vi "历史查询数据.vi"() -> ()   [LabVIEW 2019]
panel:
  out "用户名":string
  out "错误输出 2":errorcluster caption="错误输出"
  out "用户类型":string
  out "错误输出":errorcluster
  out "error out 6":errorcluster
  out "error out 5":errorcluster
  out "Row":i32
  out "Column":i32
  out "error out 7":errorcluster
  out "当前选择的记录为":string
  in  "导出文件":bool
  in  "删除记录":bool
  out "车牌查询数据":string[][](table)
  in  "返回":bool
  # "欢迎查询识别记录"
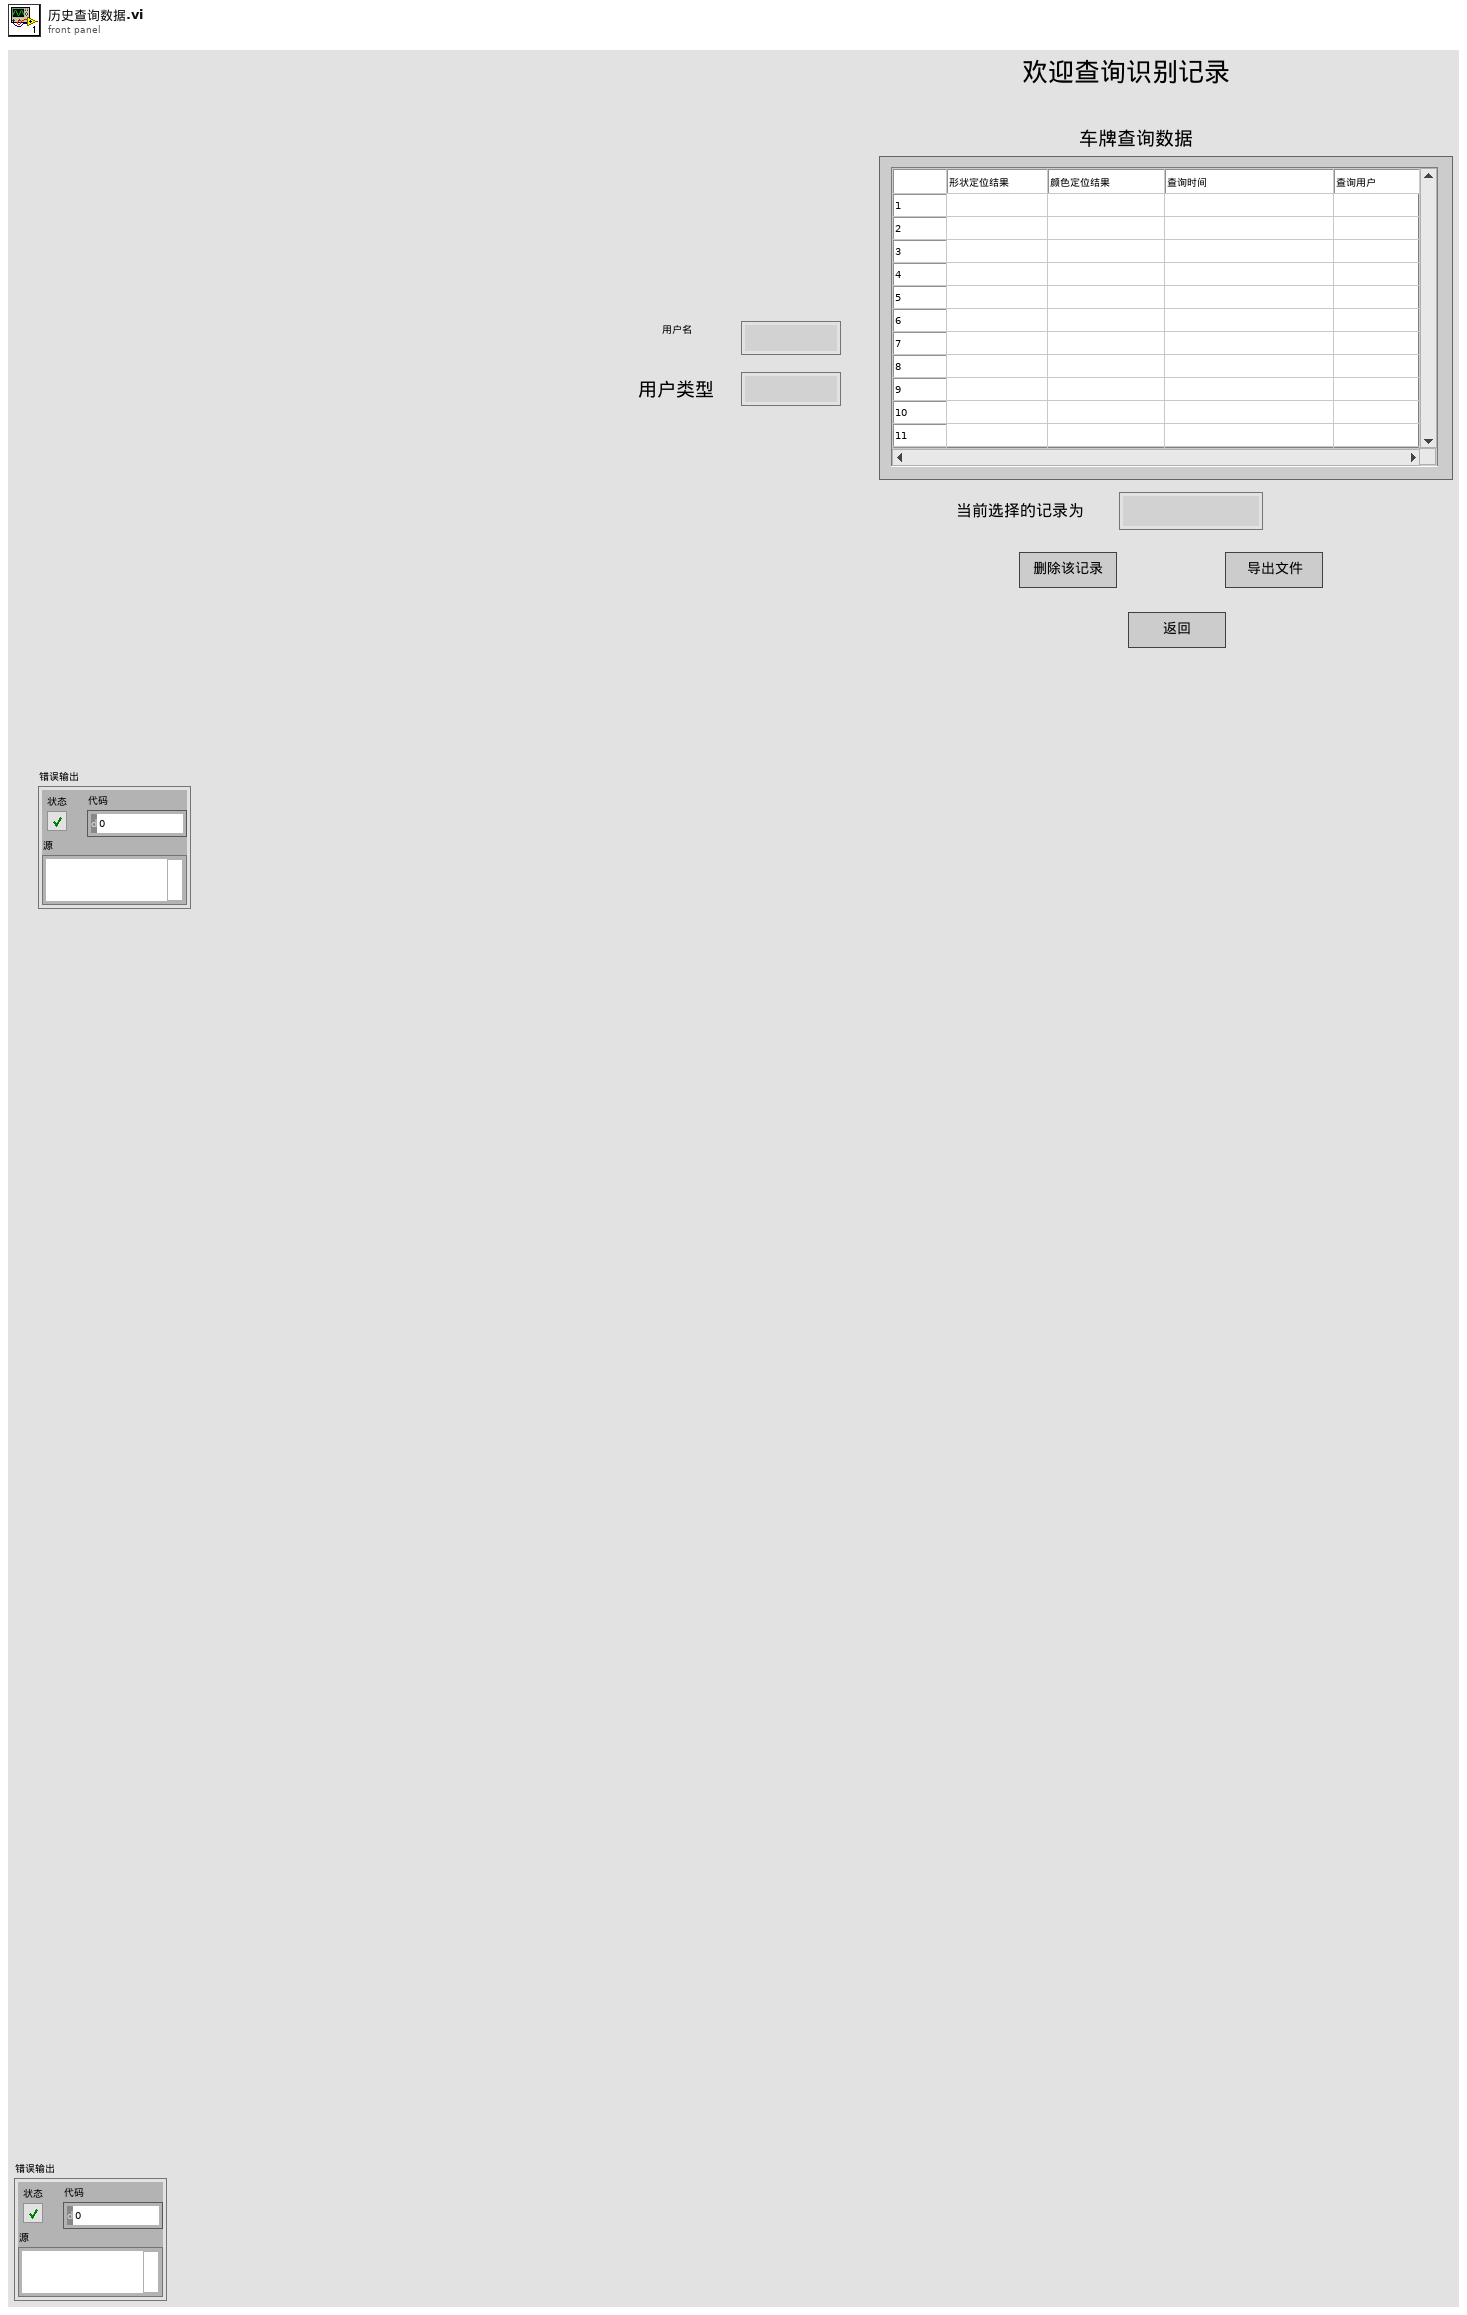
[diagram p1: front panel]
types:
  T1 = typedef "LVPoint32TypeDef.ctl" = cluster{"Horizontal":i32, "Vertical":i32}
  T2 = typedef "LVRowAndColumnTypeDef.ctl" = cluster{"Row":i32, "Column":i32}
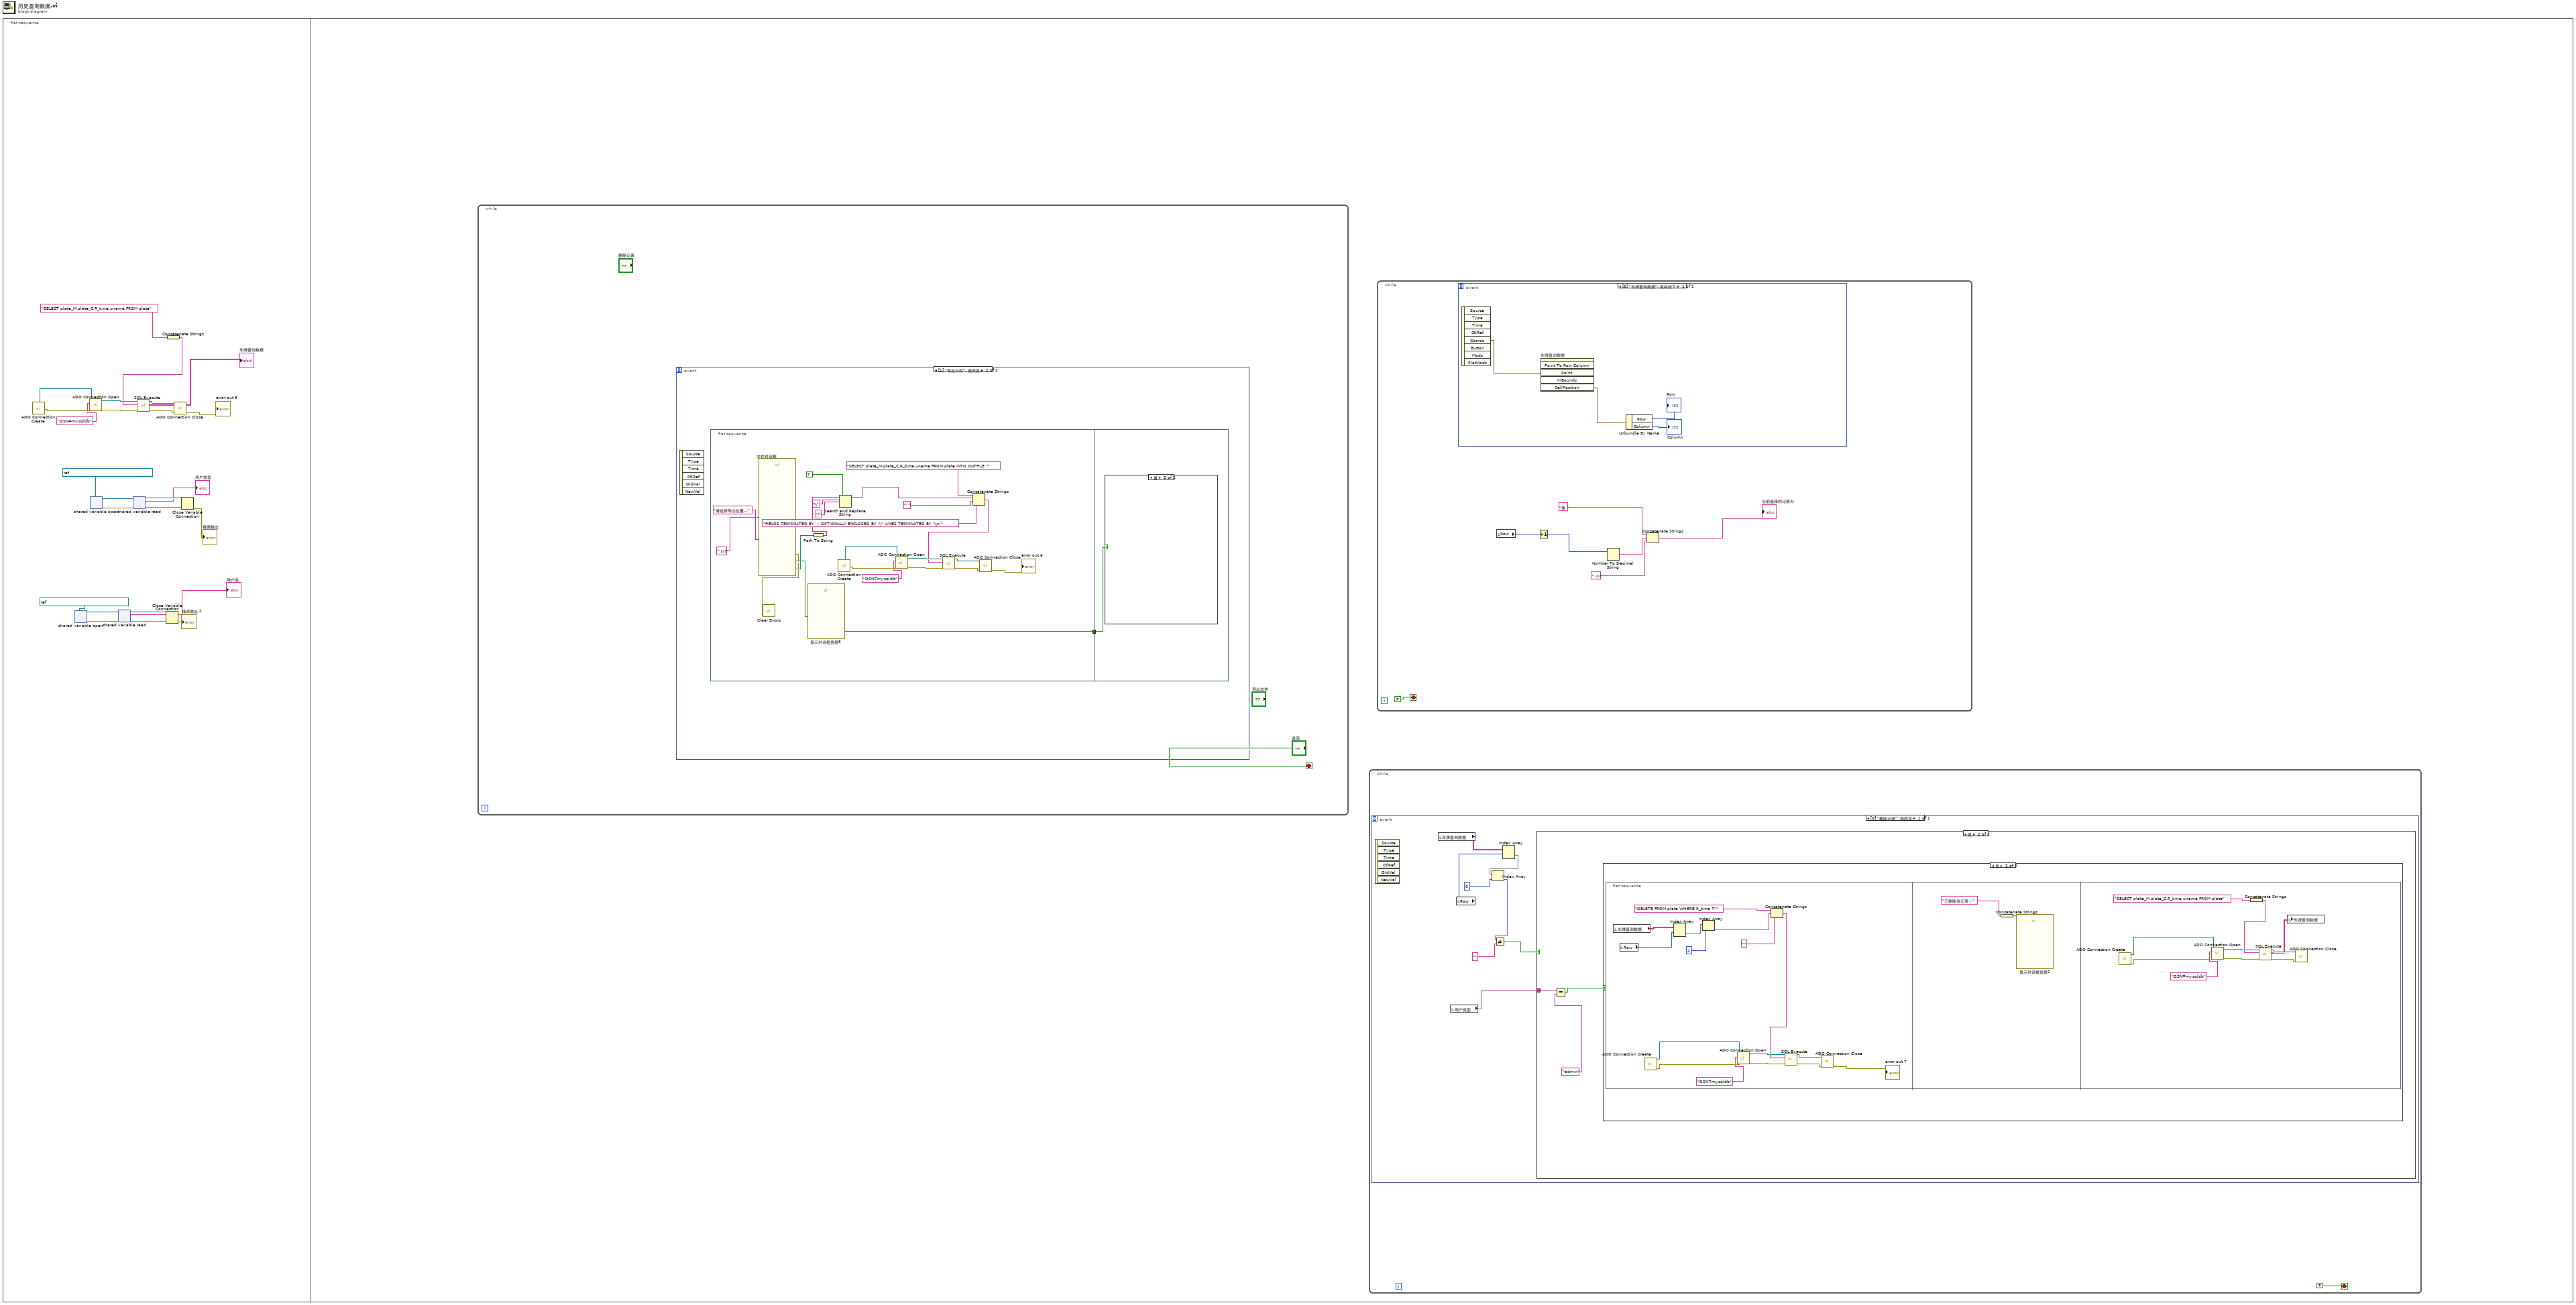
[diagram p0: block diagram]
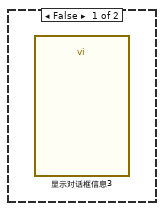
[diagram p2: hidden frame]
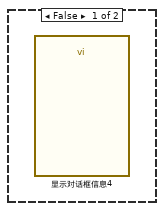
[diagram p3: hidden frame]
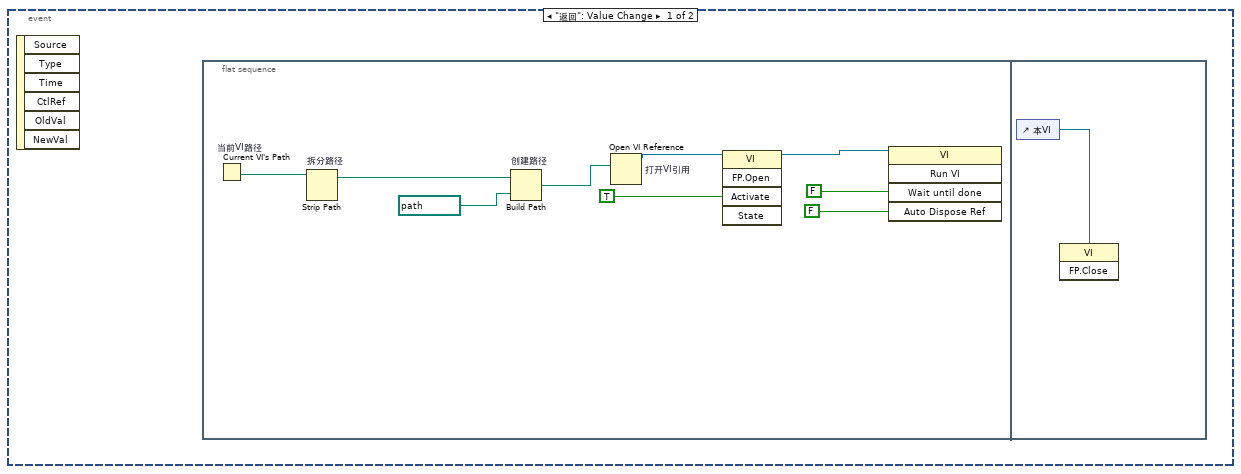
[diagram p4: hidden frame]
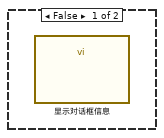
[diagram p5: hidden frame]
diagram:
  n1 = flat-sequence {
    frame #0 {
      n2 = call <userlib>:"ADO Connection Create.vi"() -> ("error out"=w20:errorcluster, "ADODB._Connection Out"=w19:refnum<k7>)  [unwired: 10 in]
      n3 = shared-variable-open(refnum<k21> "ni.var.psp://我的电脑/登录/登录用户" ("共享变量引用句柄输入")) -> (w3:refnum<k21>, w4:errorcluster)  [unwired: 2 in]
      n4 = call <userlib>:"ADO Connection Open.vi"("error in (no error)"=w20, "ConnectionString"="DSN=mysqldb", "ADODB._Connection In"=w19) -> ("error out"=w21:errorcluster, "ADODB._Connection Out"=w25:refnum<k7>)  [unwired: 7 in]
      n5 = shared-variable-open(refnum<k21> "ni.var.psp://localhost/登录/用户类型" ("共享变量引用句柄输入")) -> (w14:refnum<k21>, w13:errorcluster)  [unwired: 2 in]
      n6 = shared-variable-read(w3, w4) -> (w5:refnum<k21>, w6:errorcluster, →"用户名":string)  [unwired: 1 out]
      n7 = shared-variable-read(w14, w13) -> (w12:refnum<k21>, w11:errorcluster, →"用户类型":string)  [unwired: 1 out]
      n8 = Close Variable Connection(8:w6, 11:w5) -> (0:→"错误输出 2":errorcluster)
      n9 = Concatenate Strings("SELECT plate_M,plate_C,R_time,uname FROM plate") -> (w16:string)
      n10 = call <userlib>:"SQL Execute.vi"("error in (no error)"=w21, "Command Text"=w16, "ADODB._Connection In"=w25) -> ("error out"=w23:errorcluster, "Data"=→"车牌查询数据":string[][], "ADODB._Connection Out"=w24:refnum<k7>)  [unwired: 5 in, 1 out]
      n11 = call <userlib>:"ADO Connection Close.vi"("error in (no error)"=w23, "ADODB._Connection In"=w24) -> ("error out"=→"error out 5":errorcluster)  [unwired: 8 in, 1 out]
      n12 = Close Variable Connection(8:w11, 11:w12) -> (0:→"错误输出":errorcluster)
    }
    frame #1 {
      n13 = while {
        stop <- "返回" stop-if-true
        n14 = event shown="[1] \"导出文件\": 值改变" {
          selector: _ -> [_ _]
          dyn-events: _ -> [_ _]
          timeout: _ -> [_ _]
          event "返回": Value Change {
            n15 = event-data() -> ()  [unwired: 1 in, 6 out]
            n16 = flat-sequence {
              frame #0 {
                n17 = Current VI's Path "当前VI路径"() -> (path=w79:path)
                n18 = Strip Path "拆分路径"(path=w79) -> (stripped path=w78:path)  [unwired: 1 out]
                n19 = Build Path "创建路径"(base path=w78, name or relative path=path "登陆后.vi") -> (appended path=w81:path)
                n20 = Open VI Reference "打开VI引用"(vi path=w81) -> (vi reference=w80:refnum<vi>)  [unwired: 5 in, 1 out]
                n21 = invoke class="VI" method="FP.Open"(reference=w80, "Activate"=TRUE) -> (reference out=w84:refnum<vi>)  [unwired: 3 in, 4 out]
                n22 = invoke class="VI" method="Run VI"(reference=w84, "Wait until done"=FALSE, "Auto Dispose Ref"=FALSE) -> ()  [unwired: 2 in, 5 out]
              }
              frame #1 {
                n23 = control-ref of="本VI"() -> (w87:refnum<vi>)
                n24 = invoke class="VI" method="FP.Close"(reference=w87) -> ()  [unwired: 2 in, 3 out]
              }
            }
          }
          event "导出文件": Value Change {
            n25 = event-data() -> ()  [unwired: 1 in, 6 out]
            n26 = flat-sequence {
              tunnel: [w90] -> w88
              tunnel: w88 -> [w112]
              frame #0 {
                n27 = call "文件对话框"("prompt"="请选择导出位置...", "pattern (all files)"=".txt") -> ("selected path"=w98:path, "cancelled"=w91:bool, "error out"=w89:errorcluster)  [unwired: 10 in, 1 out]
                n28 = call <vilib>:"Clear Errors.vi"("error in (no error)"=w89) -> ()  [unwired: 5 in, 2 out]
                n29 = call "显示对话框信息5"("Enable"=w91) -> ("确定"=w90:bool)  [unwired: 9 in, 1 out]
                n30 = Path To String(path=w98) -> (string=w94:string)
                n31 = call <userlib>:"ADO Connection Create.vi"() -> ("error out"=w104:errorcluster, "ADODB._Connection Out"=w103:refnum<k7>)  [unwired: 10 in]
                n32 = Search and Replace String(replace all?=TRUE, input string=w94, search string="\\", replace string="/") -> (result string=w93:string)  [unwired: 4 in, 3 out]
                n33 = call <userlib>:"ADO Connection Open.vi"("error in (no error)"=w104, "ConnectionString"="DSN=mysqldb", "ADODB._Connection In"=w103) -> ("error out"=w105:errorcluster, "ADODB._Connection Out"=w109:refnum<k7>)  [unwired: 7 in]
                n34 = Concatenate Strings("SELECT plate_M,plate_C,R_time,uname FROM plate INTO OUTFILE '", w93, "' ", "FIELDS TERMINATED BY ',' OPTIONALLY ENCLOSED BY '\"' LINES TERMINATED BY '\\n'") -> (w100:string)
                n35 = call <userlib>:"SQL Execute.vi"("error in (no error)"=w105, "Command Text"=w100, "ADODB._Connection In"=w109) -> ("error out"=w107:errorcluster, "ADODB._Connection Out"=w108:refnum<k7>)  [unwired: 5 in, 2 out]
                n36 = call <userlib>:"ADO Connection Close.vi"("error in (no error)"=w107, "ADODB._Connection In"=w108) -> ("error out"=→"error out 6":errorcluster)  [unwired: 8 in, 1 out]
              }
              frame #1 {
                n37 = case shown="真" w112 {
                  frame False {
                    n38 = call "显示对话框信息"() -> ()  [unwired: 10 in, 2 out]
                  }
                  frame True {
                  }
                }
              }
            }
          }
        }
      }
      n39 = while {
        stop <- FALSE stop-if-true
        n40 = event shown="[0] \"删除记录\": 值改变" {
          selector: _ -> [_]
          dyn-events: _ -> [_]
          timeout: _ -> [_]
          event "删除记录": Value Change {
            n41 = event-data() -> ()  [unwired: 1 in, 6 out]
            n42 = local read "车牌查询数据"() -> (w33:string[][])
            n43 = local read "用户类型"() -> (w27:string)
            n44 = local read "Row"() -> (w32:i32)
            n45 = Index Array(array=w33, index (row)=w32) -> (element=w31:string[])  [unwired: 1 in]
            n46 = Index Array(array=w31, index=0) -> (element=w28:string)
            n47 = Not Equal?(x=w28, y="") -> (x != y?=w29:bool)
            n48 = case shown="真" w29 {
              tunnel: w27 -> [_ w37]
              frame False {
                n49 = call "显示对话框信息3"() -> ()  [unwired: 10 in, 2 out]
              }
              frame True {
                n50 = Equal?(x=w37, y="admin") -> (x = y?=w35:bool)
                n51 = case shown="真" w35 {
                  frame False {
                    n52 = call "显示对话框信息4"() -> ()  [unwired: 10 in, 2 out]
                  }
                  frame True {
                    n53 = flat-sequence {
                      frame #0 {
                        n54 = local read "车牌查询数据"() -> (w43:string[][])
                        n55 = local read "Row"() -> (w42:i32)
                        n56 = call <userlib>:"ADO Connection Create.vi"() -> ("error out"=w45:errorcluster, "ADODB._Connection Out"=w44:refnum<k7>)  [unwired: 10 in]
                        n57 = Index Array(array=w43, index (row)=w42) -> (element=w41:string[])  [unwired: 1 in]
                        n58 = Index Array(array=w41, index=2) -> (element=w39:string)
                        n59 = call <userlib>:"ADO Connection Open.vi"("error in (no error)"=w45, "ConnectionString"="DSN=mysqldb", "ADODB._Connection In"=w44) -> ("error out"=w48:errorcluster, "ADODB._Connection Out"=w52:refnum<k7>)  [unwired: 7 in]
                        n60 = Concatenate Strings("DELETE FROM plate WHERE R_time ='", w39, "'") -> (w53:string)
                        n61 = call <userlib>:"SQL Execute.vi"("error in (no error)"=w48, "Command Text"=w53, "ADODB._Connection In"=w52) -> ("error out"=w50:errorcluster, "ADODB._Connection Out"=w51:refnum<k7>)  [unwired: 5 in, 2 out]
                        n62 = call <userlib>:"ADO Connection Close.vi"("error in (no error)"=w50, "ADODB._Connection In"=w51) -> ("error out"=→"error out 7":errorcluster)  [unwired: 8 in, 1 out]
                      }
                      frame #1 {
                        n63 = Concatenate Strings("已删除该记录！") -> (w54:string)
                        n64 = call "显示对话框信息2"("Message"=w54) -> ()  [unwired: 9 in, 2 out]
                      }
                      frame #2 {
                        n65 = call <userlib>:"ADO Connection Create.vi"() -> ("error out"=w59:errorcluster, "ADODB._Connection Out"=w58:refnum<k7>)  [unwired: 10 in]
                        n66 = call <userlib>:"ADO Connection Open.vi"("error in (no error)"=w59, "ConnectionString"="DSN=mysqldb", "ADODB._Connection In"=w58) -> ("error out"=w61:errorcluster, "ADODB._Connection Out"=w64:refnum<k7>)  [unwired: 7 in]
                        n67 = Concatenate Strings("SELECT plate_M,plate_C,R_time,uname FROM plate") -> (w65:string)
                        n68 = call <userlib>:"SQL Execute.vi"("error in (no error)"=w61, "Command Text"=w65, "ADODB._Connection In"=w64) -> ("error out"=w62:errorcluster, "Data"=w56:string[][], "ADODB._Connection Out"=w63:refnum<k7>)  [unwired: 5 in, 1 out]
                        n69 = local write "车牌查询数据"(w56) -> ()
                        n70 = call <userlib>:"ADO Connection Close.vi"("error in (no error)"=w62, "ADODB._Connection In"=w63) -> ()  [unwired: 8 in, 2 out]
                      }
                    }
                  }
                }
              }
            }
          }
        }
      }
      n71 = while {
        stop <- FALSE stop-if-true
        n72 = event shown="[0] \"车牌查询数据\": 鼠标按下" {
          selector: _ -> [_]
          dyn-events: _ -> [_]
          timeout: _ -> [_]
          event "车牌查询数据": Mouse Down {
            n73 = event-data() -> ("Coords"=w76:T1)  [unwired: 1 in, 7 out]
            n74 = invoke on="车牌查询数据" class="Tbl (严格)" method="Point To Row Column"("Point"=w76) -> ("CellPosition"=w75:T2)  [unwired: 5 in, 5 out]
            n75 = Unbundle By Name(w75) -> ("Row"=→"Row":i32, "Column"=→"Column":i32)
          }
        }
        n76 = local read "Row"() -> (w67:i32)
        n77 = Increment(x=w67) -> (x+1=w66:i32)
        n78 = Number To Decimal String(number=w66) -> (decimal integer string=w70:string)  [unwired: 1 in]
        n79 = Concatenate Strings("第 ", w70, " 个") -> (→"当前选择的记录为":string)
      }
    }
  }
